vi "generate folder tree.vi"(6 "folder names[]":string[](array[string]), 8 "max length":i32, 9 "file count":i32[](array[numeric]), 11 "Size":i64[](array[numeric])) -> (3 "string":string)   [LabVIEW 2023]
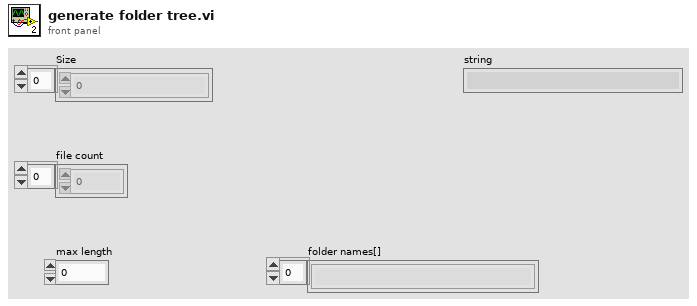
[diagram p1: front panel]
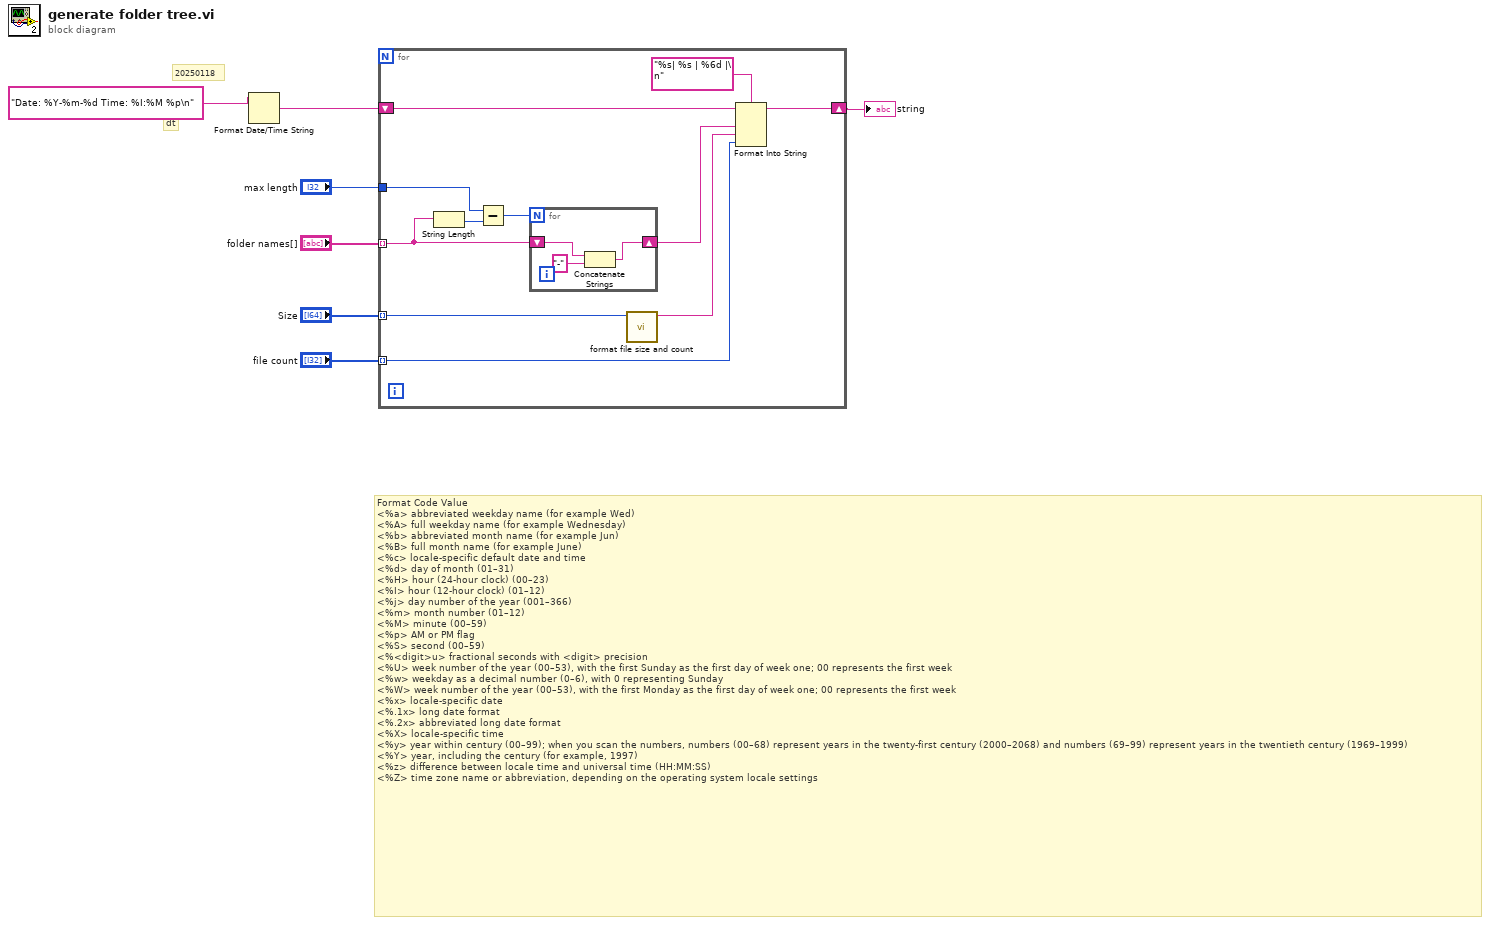
[diagram p0: block diagram]
diagram:
  # "Format Code\tValue\n<%a>\tabbreviated weekday name (for example Wed)\n<%A>\tfull weekday name (for example Wednesday)\n<%b>\tabbreviated month name (for example Jun)\n<%B>\tfull month name (for example June)\n<%c>\tlocale-specific default date and time\n<%d>\tday of month (01–31)\n<%H>\thour (24-hour clock) (00–23)\n<%I>\thour (12-hour clock) (01–12)\n<%j>\tday number of the year (001–366)\n<%m>\tmonth number (01–12)\n<%M>\tminute (00–59)\n<%p>\tAM or PM flag\n<%S>\tsecond (00–59)\n<%<digit>u>\tfractional seconds with <digit> precision\n<%U>\tweek number of the year (00–53), with the first Sunday as the first day of week one; 00 represents the first week\n<%w>\tweekday as a decimal number (0–6), with 0 representing Sunday\n<%W>\tweek number of the year (00–53), with the first Monday as the first day of week one; 00 represents the first week\n<%x>\tlocale-specific date\n<%.1x>\tlong date format\n<%.2x>\tabbreviated long date format\n<%X>\tlocale-specific time\n<%y>\tyear within century (00–99); when you scan the numbers, numbers (00–68) represent years in the twenty-first century (2000–2068) and numbers (69–99) represent years in the twentieth century (1969–1999)\n<%Y>\tyear, including the century (for example, 1997)\n<%z>\tdifference between locale time and universal time (HH:MM:SS)\n<%Z>\ttime zone name or abbreviation, depending on the operating system locale settings"
  # "dt"
  # "20250118"
  n1 = Format Date/Time String(time format string (%c)="Date: %Y-%m-%d Time: %I:%M %p\n") -> (date/time string=w2:string)  [unwired: 2 in]
  n2 = for {
    tunnel: "Size" -> [w14] mode=indexing
    tunnel: "file count" -> [w9] mode=indexing
    tunnel: "folder names[]" -> [w15] mode=indexing
    tunnel: "max length" -> [w18]
    shift-right: [w12] -> w3
    shift-left: w2 -> [w13]
    n3 = String Length(string=w15) -> (length=w17:i32)
    n4 = Subtract(x=w18, y=w17) -> (x-y=w16:i32)
    n5 = for {
      N: w16 -> [_]
      shift-right: [w20] -> w11
      shift-left: w15 -> [w21]
      n6 = Concatenate Strings(w21, "-" ("string")) -> (w20:string)
    }
    n7 = call "format file size and count.vi"("size"=w14) -> ("size"=w10:string)  [unwired: 10 in]
    n8 = Format Into String(format string="%s| %s | %6d |\n", initial string=w13, w11, w10, w9) -> (resulting string=w12:string)  [unwired: 1 in, 1 out]
  }
  "string" <- w3
